vi "Flussdichte_Anpassen.vi"(0 "VISA Name FG in (FG)":refnum<visa-resource-name>="USB0::0x0957::0x0407::MY44043889::INSTR", 1 "VISA Name OZ In (OZ)":refnum<visa-resource-name>="USB0::0x0957::0x179B::MY54313507::INSTR", 2 "Querschnitt A":dbl=45.0 format="%#_13g", 3 "b_gew":dbl=1.0 format="%#_13g", 4 "Anzahl_Messpunkte":i32=8000, 5 "Faktor1":dbl=31.0 format="%#_13g", 6 "Faktor2":dbl=744.0 format="%#_13g", 7 "Error_in":errorcluster, 8 "min Spg FG":dbl=0.2 format="%#_13g", 10 "max Spg FG":dbl=20.0 format="%#_13g") -> (13 "bmin1":dbl, 15 "hmin1":dbl, 17 "hmax1":dbl, 19 "hmax2":dbl, 20 "VISA Name FG out":refnum<visa-resource-name>="USB0::0x0957::0x0407::MY44043889::INSTR", 21 "VISA Name OZ Out":refnum<visa-resource-name>="USB0::0x0957::0x179B::MY54313507::INSTR", 22 "b_gew":dbl, 23 "spg_abw":dbl format="%#_13g", 24 "spg":dbl, 25 "add":dbl, 27 "Error_out":errorcluster)   [LabVIEW 2016]
doc: "Übergibt dem VI Anpassung die Spannungswerte. Die Spannungswerte werden in 2V, 1V, 0,5V, 0,1V, 0,05V, 0,02V Schritten an das VI übergeben.\n\nBricht den Vorgang ab sobald die gewünschte Spannung erreicht wird und gibt diese weiter. Es werden außerdem noch die gewünschte Flussdichte ausgegeben."
panel:
  out "bmax1":dbl
  in  "GUI data":T1
  in  "GUI Einstellungen":T2
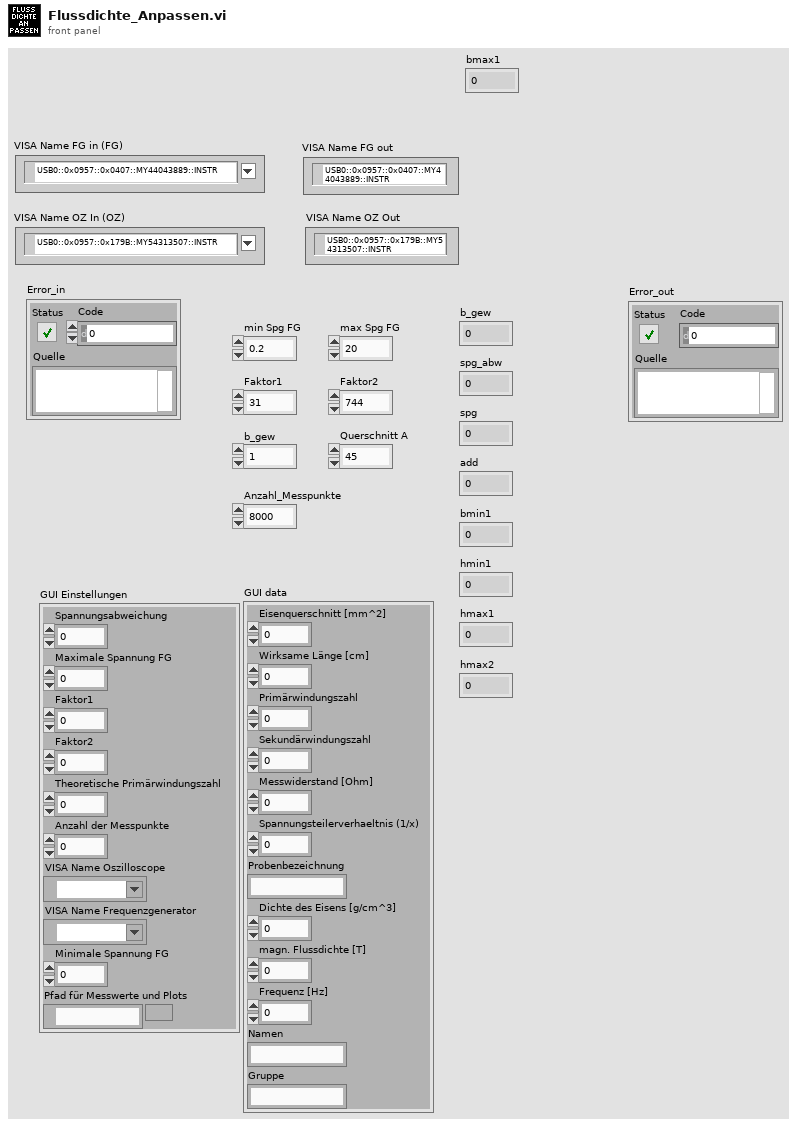
[diagram p1: front panel]
types:
  T1 = cluster{"Eisenquerschnitt [mm^2]":dbl, "Wirksame Länge [cm]":dbl, "Primärwindungszahl":dbl, "Sekundärwindungszahl":dbl, "Messwiderstand [Ohm]":dbl, "Spannungsteilerverhaeltnis (1/x)":dbl, "Probenbezeichnung":string, "Dichte des Eisens [g/cm^3]":dbl, "magn. Flussdichte [T]":dbl, "Frequenz [Hz]":dbl, "Namen":string, "Gruppe":string}
  T2 = cluster{"Spannungsabweichung":dbl, "Maximale Spannung FG":dbl, "Faktor1":dbl, "Faktor2":dbl, "Theoretische Primärwindungszahl":dbl, "Anzahl der Messpunkte":i32, "VISA Name Oszilloscope":refnum<visa-resource-name>, "VISA Name Frequenzgenerator":refnum<visa-resource-name>, "Minimale Spannung FG":dbl, "Pfad für Messwerte und Plots":path}
  T3 = enum16{"Add_2V", "Add_1V", "Add_0.5V", "Add_0.1V", "Add_0.05V", "Add_0.02V", ""}
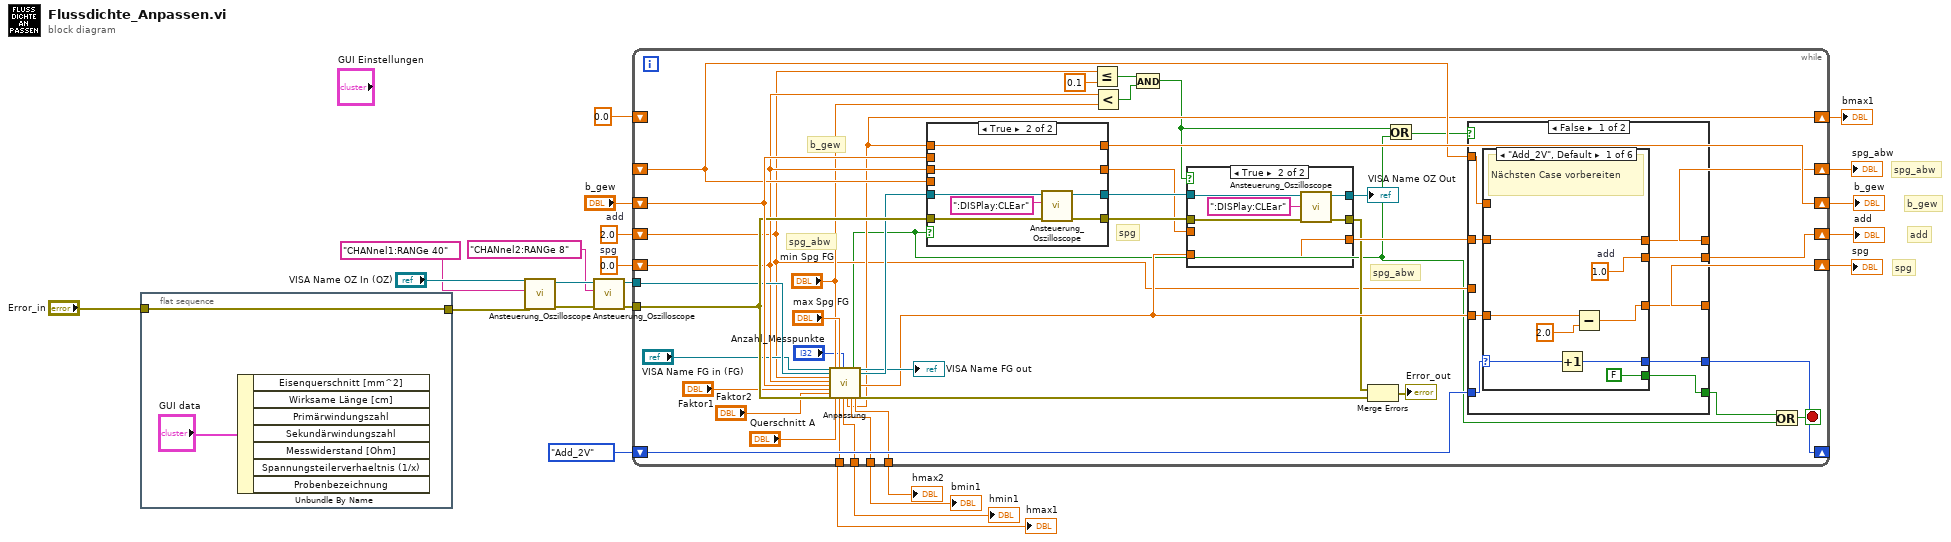
[diagram p0: block diagram]
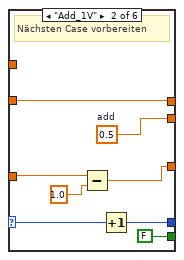
[diagram p2: hidden frame]
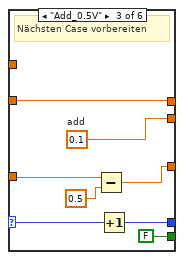
[diagram p3: hidden frame]
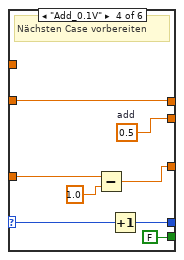
[diagram p4: hidden frame]
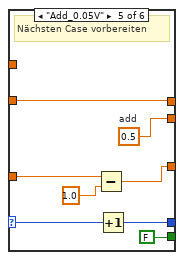
[diagram p5: hidden frame]
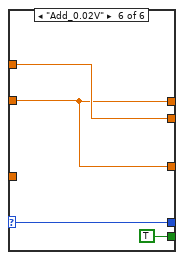
[diagram p6: hidden frame]
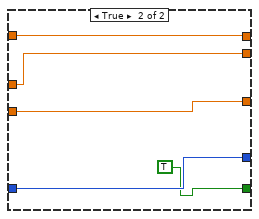
[diagram p7: hidden frame]
diagram:
  w16 = 0.0  # spg
  w17 = 2.0  # add
  # "b_gew"
  # "spg_abw"
  # "add"
  # "spg"
  n1 = flat-sequence {
    tunnel: "Error_in" -> [w24]
    tunnel: [w24] -> w3
    frame #0 {
      n2 = Unbundle By Name("GUI data") -> ()  [unwired: 7 out]
    }
  }
  n3 = call "Ansteuerung_Oszilloscope.vi"("Error_in"=w3, "Eingangs-String"="CHANnel1:RANGe 40", "VISA Name OZ in(OZ)"="VISA Name OZ In (OZ)") -> ("Error_out"=w20:errorcluster, "VISA Name OZ out"=w21:refnum<visa-resource-name>)  [unwired: 6 in, 1 out]
  n4 = call "Ansteuerung_Oszilloscope.vi"("Error_in"=w20, "Eingangs-String"="CHANnel2:RANGe 8", "VISA Name OZ in(OZ)"=w21) -> ("Error_out"=w13:errorcluster, "VISA Name OZ out"=w14:refnum<visa-resource-name>)  [unwired: 6 in, 1 out]
  n5 = while {
    shift-right: [w67] -> _
    shift-left: T3."Add_2V" -> [w68]
    shift-right: [w66] -> w6
    shift-left: w17 -> [w28]
    shift-right: [w65] -> w5
    shift-left: w16 -> [w52]
    shift-right: [w64] -> w7
    shift-left: "b_gew" -> [w63]
    shift-right: [w50] -> w12
    shift-left: _ -> [w54]
    tunnel: w14 -> [w61]
    tunnel: w13 -> [w62]
    tunnel: [w36] -> w11
    tunnel: [w35] -> w10
    tunnel: [w34] -> w9
    tunnel: [w33] -> w8
    shift-right: [w31] -> w1
    shift-left: 0.0 -> [_]
    stop <- w42 stop-if-true
    # "spg_abw"
    # "spg_abw"
    # "spg"
    # "b_gew"
    n6 = call "Anpassung.vi"("VISA Name FG in(FG)"="VISA Name FG in (FG)", "VISA Name OZ In (OZ)"=w61, "Add (0)"=w28, "Spg (0)"=w52, "b_gew"=w63, "Faktor1"="Faktor1", "Faktor2"="Faktor2", "Error_in"=w62, "min Spg FG"="min Spg FG", "Querschnitt A"="Querschnitt A", "max Spg FG"="max Spg FG", "Anzahl_Messpunkte"="Anzahl_Messpunkte") -> ("hmax1"=w36:dbl, "hmin1"=w35:dbl, "bmax1"=w31:dbl, "bmin1"=w34:dbl, "Abbruch (VI verlassen) = merker1"=w26:bool, "hmax2"=w33:dbl, "VISA Name FG out"=→"VISA Name FG out":refnum<visa-resource-name>, "VISA Name OZ Out"=w60:refnum<visa-resource-name>, "spg"=w43:dbl, "Error_out"=w38:errorcluster)  [unwired: 1 in, 5 out]
    n7 = case shown="True" w26 {
      tunnel: w31 -> [_ w146]
      tunnel: [w137 w146] -> w64
      tunnel: w63 -> [w137 _]
      tunnel: w52 -> [_ w145]
      tunnel: [w136 w145] -> w53
      tunnel: w54 -> [w136 _]
      tunnel: w60 -> [w139 w143]
      tunnel: w62 -> [w138 w142]
      tunnel: [w139 w141] -> w56
      tunnel: [w138 w140] -> w55
      frame False {
      }
      frame True {
        n8 = call "Ansteuerung_Oszilloscope.vi"("Error_in"=w142, "Eingangs-String"=":DISPlay:CLEar", "VISA Name OZ in(OZ)"=w143) -> ("Error_out"=w140:errorcluster, "VISA Name OZ out"=w141:refnum<visa-resource-name>)  [unwired: 6 in, 1 out]
      }
    }
    n9 = Less Or Equal?(x=w28, y=0.1) -> (x <= y?=w58:bool)
    n10 = Less?(x=w52, y="min Spg FG") -> (x < y?=w57:bool)
    n11 = And(x=w58, y=w57) -> (x .and. y?=w29:bool)
    n12 = case shown="True" w29 {
      tunnel: w56 -> [w128 w134]
      tunnel: w55 -> [w127 w133]
      tunnel: w53 -> [w129 _]
      tunnel: w43 -> [_ w132]
      tunnel: [w129 w132] -> w51
      tunnel: [w128 w131] -> w44
      tunnel: [w127 w130] -> w39
      frame False {
      }
      frame True {
        n13 = call "Ansteuerung_Oszilloscope.vi"("Error_in"=w133, "Eingangs-String"=":DISPlay:CLEar", "VISA Name OZ in(OZ)"=w134) -> ("Error_out"=w130:errorcluster, "VISA Name OZ out"=w131:refnum<visa-resource-name>)  [unwired: 6 in, 1 out]
      }
    }
    "VISA Name OZ Out" <- w44
    n14 = Merge Errors(w39, w38) -> (→"Error_out":errorcluster)
    n15 = Or(x=w29, y=w26) -> (x .or. y?=w30:bool)
    n16 = case shown="False" w30 {
      tunnel: w68 -> [w70 w123]
      tunnel: [w77 w123] -> w67
      tunnel: [w76 w124] -> w66
      tunnel: [w75 w125] -> w65
      tunnel: w54 -> [w74 _]
      tunnel: w51 -> [w73 w126]
      tunnel: [w72 w126] -> w50
      tunnel: w43 -> [w71 w125]
      tunnel: [w69 TRUE] -> w27
      tunnel: w28 -> [_ w124]
      frame False {
        n17 = case shown="\"Add_2V\", Default" w70 {
          selector: w70 -> [w85 w93 w101 w109 w117 w121]
          tunnel: [w84 w92 w100 w108 w116 w121] -> w77
          tunnel: [w83 w88 w96 w104 w112 w119] -> w76
          tunnel: [w81 w89 w97 w105 w113 w118] -> w75
          tunnel: w71 -> [w80 w90 w98 w106 w114 _]
          tunnel: [FALSE FALSE FALSE FALSE FALSE TRUE] -> w69
          tunnel: w74 -> [_ _ _ _ _ w119]
          tunnel: w73 -> [w79 w87 w95 w103 w111 w118]
          tunnel: [w79 w87 w95 w103 w111 w118] -> w72
          frame "Add_2V", Default {
            w83 = 1.0  # add
            # "Nächsten Case vorbereiten"
            n18 = Increment(x=w85) -> (x+1=w84:T3)
            n19 = Subtract(x=w80, y=2.0 ("spg")) -> (x-y=w81:dbl)
          }
          frame "Add_1V" {
            w88 = 0.5  # add
            # "Nächsten Case vorbereiten"
            n20 = Subtract(x=w90, y=1.0 ("spg")) -> (x-y=w89:dbl)
            n21 = Increment(x=w93) -> (x+1=w92:T3)
          }
          frame "Add_0.5V" {
            w96 = 0.1  # add
            # "Nächsten Case vorbereiten"
            n22 = Subtract(x=w98, y=0.5 ("spg")) -> (x-y=w97:dbl)
            n23 = Increment(x=w101) -> (x+1=w100:T3)
          }
          frame "Add_0.1V" {
            w104 = 0.5  # add
            # "Nächsten Case vorbereiten"
            n24 = Subtract(x=w106, y=1.0 ("spg")) -> (x-y=w105:dbl)
            n25 = Increment(x=w109) -> (x+1=w108:T3)
          }
          frame "Add_0.05V" {
            w112 = 0.5  # add
            # "Nächsten Case vorbereiten"
            n26 = Subtract(x=w114, y=1.0 ("spg")) -> (x-y=w113:dbl)
            n27 = Increment(x=w117) -> (x+1=w116:T3)
          }
          frame "Add_0.02V" {
          }
        }
      }
      frame True {
      }
    }
    n28 = Or(x=w27, y=w26) -> (x .or. y?=w42:bool)
  }
  "spg_abw" <- w12
  "hmax1" <- w11
  "hmin1" <- w10
  "bmin1" <- w9
  "hmax2" <- w8
  "b_gew" <- w7
  "add" <- w6
  "spg" <- w5
  "bmax1" <- w1
